vi "Configure IQ Output.vi"(0 "VISA resource name":refnum<visa-resource-name>, 1 "External Filter (1: Through)":u16(ring)=1 items=["40 MHz", "Through"], 2 "Enable Automatic External Filter (T:Enable)":bool=TRUE, 5 "Modulation Format (1: Dual Modulation)":u16(ring)=1 items=["Dual Modulation"=1, "Dual ARB"=2, "Multitone"=3, "Digital Modulation"=4, "Two-tone"=6, "AWGN Real-Time"=7, "AWGN ARB"=8], 7 "I/Q Attenuation Auto Mode (T:Enable)":bool=TRUE, 9 "I/Q Attenuation Level (2 dB)":dbl=2.0, 11 "error in (no error)":errorcluster, 12 "Enable Automatic Modulation Filter (T:Enable)":bool=TRUE, 13 "Modulation Filter (2: Through)":u16(ring)=2 items=["2.1 MHz", "40 MHz", "Through"]) -> (4 "VISA resource name out":refnum<visa-resource-name>, 15 "error out":errorcluster)   [LabVIEW 2011, in "Agilent PSG MXG Series.lvlib"]
doc: "Configures I/Q attenuation, external filter and modulation filter.\n\n<B>Notes:</B>\n(1) This VI is valid only in E8267C, E8257D, E8267D, N5182A.\n\n(2) For E8267C, this VI is valid only when the instrument installs <B>Option 002</B> (Internal baseband generator) or <B>Option 602</B> (Digital bus baseband generator).\n\n(3) For E8267D, this VI is valid only when the instrument installs <B>Option 601</B> or <B>Option 602</B> (Internal baseband generator).\n\n(4) For N5182A, this VI is valid only when the instrument installs <B>Option 651</B> or <B>Option 652</B> or <B>Option 654</B> (Internal baseband generator)."
uses:
  Agilent PSG MXG Series.lvlib
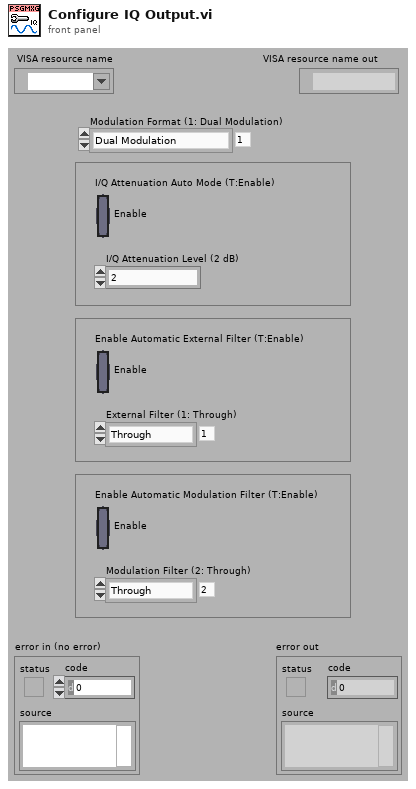
[diagram p1: front panel]
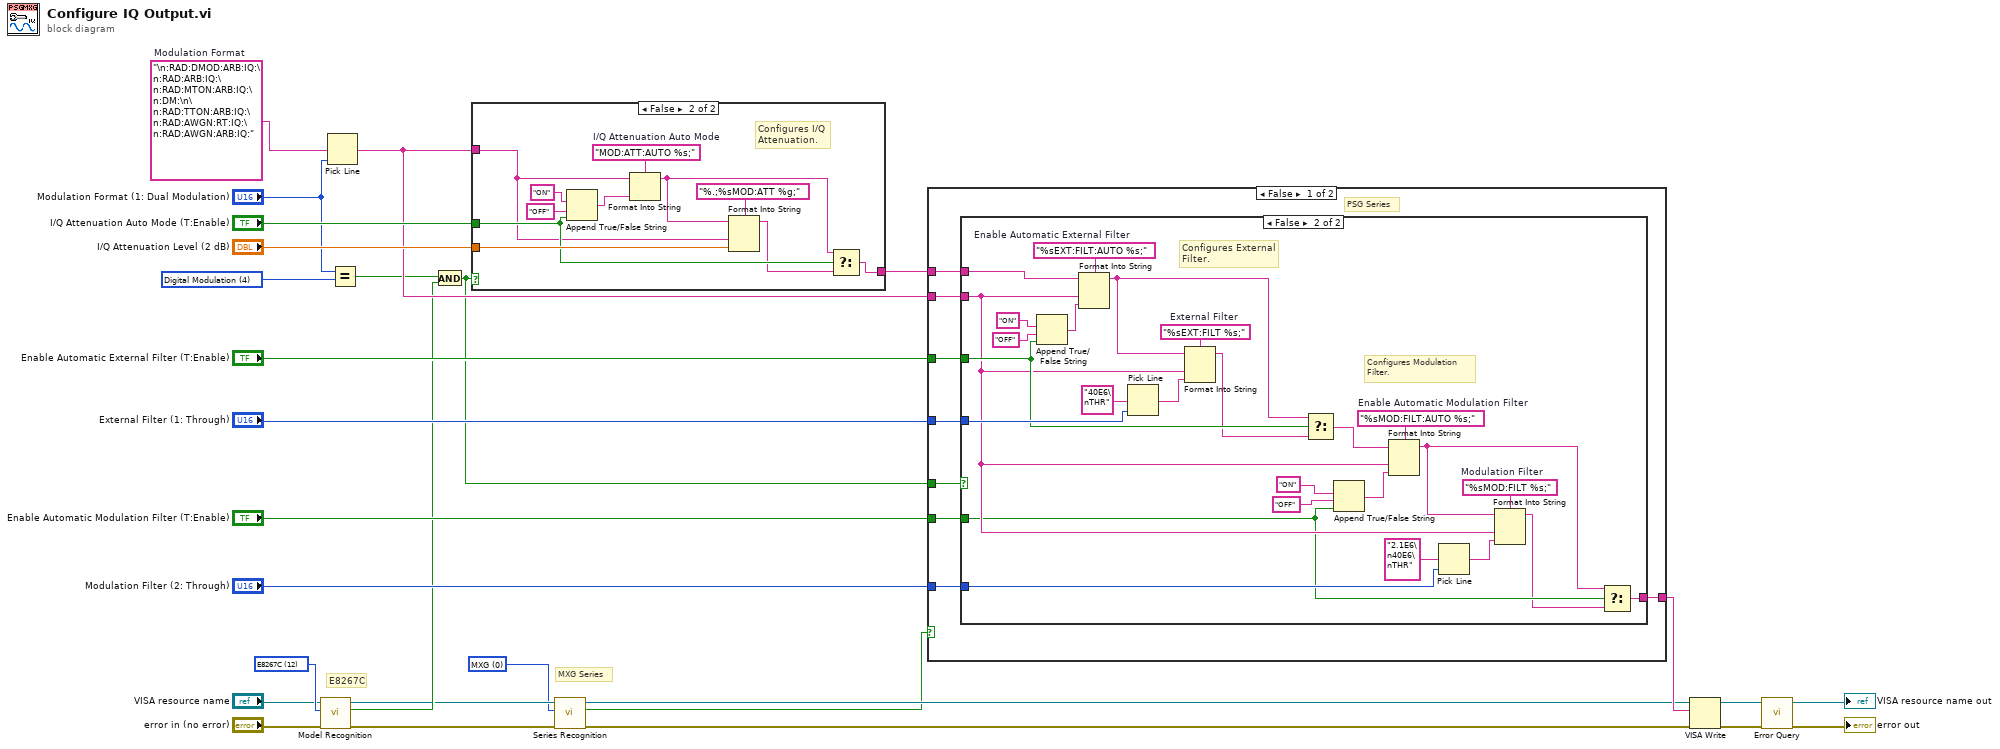
[diagram p0: block diagram]
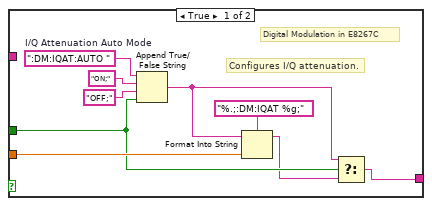
[diagram p2: hidden frame]
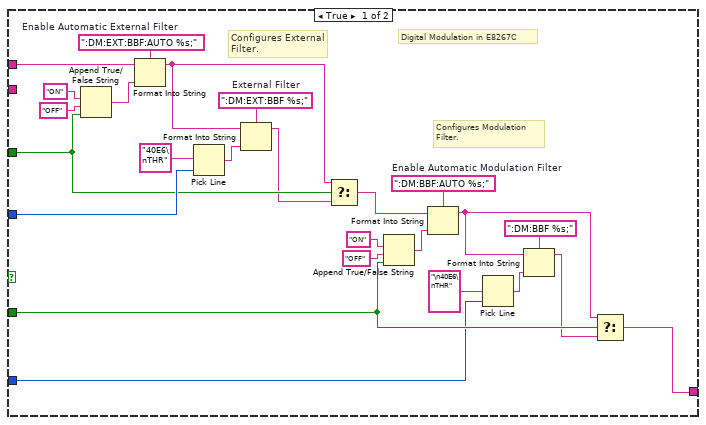
[diagram p3: hidden frame]
diagram:
  w7 = u16 0 items=["MXG", "PSG", "PSG-A", "PSG-C", "PSG-D"] ("Series Type (0: MXG)")
  w13 = u16 12 items=["N5181A"=0, "N5182A"=1, "E8241A"=5, "E8244A"=6, "E8251A"=7, "E8254A"=8, "E8247C"=10, "E8257C"=11, "E8267C"=12, "E8257D"=15, "E8267D"=16] ("Model Type (0: N5181A)")
  w16 = u16 4 items=["Dual Modulation"=1, "Dual ARB"=2, "Multitone"=3, "Digital Modulation"=4] ("Format (1: Dual Modulation)")
  w28 = "\n:RAD:DMOD:ARB:IQ:\n:RAD:ARB:IQ:\n:RAD:MTON:ARB:IQ:\n:DM:\n\n:RAD:TTON:ARB:IQ:\n:RAD:AWGN:RT:IQ:\n:RAD:AWGN:ARB:IQ:"  # Modulation Format
  # "E8267C"
  # "MXG Series"
  n1 = call "Model Recognition.vi"("error in (no error)"="error in (no error)", "Model Type (0: N5181A)"=w13, "VISA resource name"="VISA resource name") -> ("error out"=w8:errorcluster, "Is Model Correct"=w12:bool, "VISA resource name out"=w9:refnum<visa-resource-name>)  [unwired: 6 in]
  n2 = Pick Line(multi-line string=w28, line index="Modulation Format (1: Dual Modulation)") -> (output string=w25:string)  [unwired: 1 in]
  n3 = Equal?(x="Modulation Format (1: Dual Modulation)", y=w16) -> (x = y?=w15:bool)
  n4 = And(x=w15, y=w12) -> (x .and. y?=w5:bool)
  n5 = case shown="False" w5 {
    tunnel: "I/Q Attenuation Level (2 dB)" -> [w34 w43]
    tunnel: "I/Q Attenuation Auto Mode (T:Enable)" -> [w32 w42]
    tunnel: w25 -> [_ w39]
    tunnel: [w29 w38] -> w24
    frame True {
      w37 = ":DM:IQAT:AUTO "  # I/Q Attenuation Auto Mode
      # "Configures I/Q attenuation."
      # "Digital Modulation in E8267C"
      n6 = Append True/False String(1:w32, 2:"OFF;" ("false string"), 3:"ON;" ("true string"), 4:w37) -> (0:w30:string)
      n7 = Format Into String(format string="%.;:DM:IQAT %g;", initial string=w30, w34) -> (resulting string=w31:string)  [unwired: 1 in, 1 out]
      n8 = Select(t=w30, s=w32, f=w31) -> (s? t:f=w29:string)
    }
    frame False {
      w48 = "MOD:ATT:AUTO %s;"  # I/Q Attenuation Auto Mode
      # "Configures I/Q\nAttenuation."
      n9 = Append True/False String(1:w42, 2:"OFF" ("false string"), 3:"ON" ("true string")) -> (0:w47:string)  [unwired: 1 in]
      n10 = Format Into String(format string=w48, initial string=w39, w47) -> (resulting string=w40:string)  [unwired: 1 in, 1 out]
      n11 = Format Into String(format string="%.;%sMOD:ATT %g;", initial string=w40, w39, w43) -> (resulting string=w41:string)  [unwired: 1 in, 1 out]
      n12 = Select(t=w40, s=w42, f=w41) -> (s? t:f=w38:string)
    }
  }
  n13 = call "Series Recognition.vi"("error in (no error)"=w8, "Series Type (0: MXG)"=w7, "VISA resource name"=w9) -> ("error out"=w10:errorcluster, "Is Series Correct"=w6:bool, "VISA resource name out"=w11:refnum<visa-resource-name>)  [unwired: 6 in]
  n14 = case shown="False" w6 {
    tunnel: w25 -> [w53 _]
    tunnel: w24 -> [w56 w108]
    tunnel: "Enable Automatic External Filter (T:Enable)" -> [w54 _]
    tunnel: "External Filter (1: Through)" -> [w55 _]
    tunnel: "Enable Automatic Modulation Filter (T:Enable)" -> [w51 _]
    tunnel: "Modulation Filter (2: Through)" -> [w52 _]
    tunnel: [w50 w108] -> w19
    tunnel: w5 -> [w49 _]
    frame False {
      # "PSG Series"
      n15 = case shown="False" w49 {
        tunnel: w56 -> [w81 w106]
        tunnel: w55 -> [w73 w99]
        tunnel: w54 -> [w72 w98]
        tunnel: w53 -> [_ w89]
        tunnel: w52 -> [w60 w86]
        tunnel: w51 -> [w63 w85]
        tunnel: [w57 w82] -> w50
        frame True {
          w68 = ":DM:BBF:AUTO %s;"  # Enable Automatic Modulation Filter
          w76 = ":DM:EXT:BBF %s;"  # External Filter
          w80 = ":DM:EXT:BBF:AUTO %s;"  # Enable Automatic External Filter
          # "Configures Modulation\nFilter."
          # "Configures External\nFilter."
          # "Digital Modulation in E8267C"
          n16 = Append True/False String(1:w72, 2:"OFF" ("false string"), 3:"ON" ("true string")) -> (0:w79:string)  [unwired: 1 in]
          n17 = Format Into String(format string=w80, initial string=w81, w79) -> (resulting string=w70:string)  [unwired: 1 in, 1 out]
          n18 = Pick Line(multi-line string="40E6\nTHR", line index=w73) -> (output string=w75:string)  [unwired: 1 in]
          n19 = Format Into String(format string=w76, initial string=w70, w75) -> (resulting string=w71:string)  [unwired: 1 in, 1 out]
          n20 = Select(t=w70, s=w72, f=w71) -> (s? t:f=w69:string)
          n21 = Append True/False String(1:w63, 2:"OFF" ("false string"), 3:"ON" ("true string")) -> (0:w67:string)  [unwired: 1 in]
          n22 = Format Into String(format string=w68, initial string=w69, w67) -> (resulting string=w58:string)  [unwired: 1 in, 1 out]
          n23 = Pick Line(multi-line string="\n40E6\nTHR", line index=w60) -> (output string=w61:string)  [unwired: 1 in]
          n24 = Format Into String(format string=":DM:BBF %s;", initial string=w58, w61) -> (resulting string=w59:string)  [unwired: 1 in, 1 out]
          n25 = Select(t=w58, s=w63, f=w59) -> (s? t:f=w57:string)
        }
        frame False {
          w90 = "%sMOD:FILT %s;"  # Modulation Filter
          w94 = "%sMOD:FILT:AUTO %s;"  # Enable Automatic Modulation Filter
          w102 = "%sEXT:FILT %s;"  # External Filter
          w107 = "%sEXT:FILT:AUTO %s;"  # Enable Automatic External Filter
          # "Configures Modulation\nFilter."
          # "Configures External\nFilter."
          n26 = Append True/False String(1:w98, 2:"OFF" ("false string"), 3:"ON" ("true string")) -> (0:w103:string)  [unwired: 1 in]
          n27 = Format Into String(format string=w107, initial string=w106, w89, w103) -> (resulting string=w96:string)  [unwired: 1 in, 1 out]
          n28 = Pick Line(multi-line string="40E6\nTHR", line index=w99) -> (output string=w101:string)  [unwired: 1 in]
          n29 = Format Into String(format string=w102, initial string=w96, w89, w101) -> (resulting string=w97:string)  [unwired: 1 in, 1 out]
          n30 = Select(t=w96, s=w98, f=w97) -> (s? t:f=w95:string)
          n31 = Append True/False String(1:w85, 2:"OFF" ("false string"), 3:"ON" ("true string")) -> (0:w93:string)  [unwired: 1 in]
          n32 = Format Into String(format string=w94, initial string=w95, w89, w93) -> (resulting string=w83:string)  [unwired: 1 in, 1 out]
          n33 = Pick Line(multi-line string="2.1E6\n40E6\nTHR", line index=w86) -> (output string=w88:string)  [unwired: 1 in]
          n34 = Format Into String(format string=w90, initial string=w83, w89, w88) -> (resulting string=w84:string)  [unwired: 1 in, 1 out]
          n35 = Select(t=w83, s=w85, f=w84) -> (s? t:f=w82:string)
        }
      }
    }
    frame True {
      # "N5182A"
    }
  }
  n36 = VISA Write(VISA resource name=w11, write buffer=w19, error in (no error)=w10) -> (VISA resource name out=w18:refnum<visa-resource-name>, error out=w17:errorcluster)  [unwired: 1 out]
  n37 = call "Error Query.vi"("error in (no error)"=w17, "VISA resource name"=w18) -> ("error out"=→"error out":errorcluster, "VISA resource name out"=→"VISA resource name out":refnum<visa-resource-name>)  [unwired: 6 in, 2 out]
